vi "CSV_Setup_Data_Handler_2.0.vi"(0 "first iteration":bool, 1 "Timeout 1":bool, 7 "Sample Data":dbl[](array[numeric]), 9 "Sample Data 2":dbl[](array[numeric]), 11 "Data":T1={"Camera 1"={"Camera1"="", "Cam 1"=FALSE, "CAM1 Model"=enum."a2A5328-15ucBAS", "Cam1 ID"=0}, "Camera 2"={"Camera2"="", "Cam 2"=FALSE, "CAM2 Model"=enum."a2A5328-15ucBAS", "Cam2 ID"=0}, "Image"={"Camera1_Img"=refnum, "Camera2_Img"=refnum, "Img1_Orig_Disp"=refnum, "Img2_Orig_Disp"=refnum, "Img1_Orig_RGB"=refnum, "Img2_Orig_RGB"=refnum, "Blue_Plane_Extract"=refnum, "Subtracted_Plane"=refnum, "Img1_Binary"=refnum, "Img2_Binary"=refnum, "Crop_Mask"=refnum, "Img1_Save"=refnum, "Img2_Save"=refnum, "Img1_Cali_Full"=refnum, "Img2_Cali_Full"=refnum, "Img1_Cali_Detect"=refnum, "Img2_Cali_Detect"=refnum}, "Ques"={"Cam 1 queue"=refnum, "Cam 2 queue"=refnum, "Cam 1 - save queue"=refnum, "Cam 2 - save queue"=refnum, "Image Process Queue Size"=500, "Image Save Queue Size"=500, "Overload threshold"=500, "Max large object threshold"=0}, "Arduino SRS"={"Pinch-valve"="", "Actuator"=FALSE, "Arduino Uno"="", "Valve state"=enum."Open"}, "Pump"={"Port"="", "Connection"=FALSE, "Flush Size"=0, "Command"="", "Pump Size"=enum."Large", "Pump"="", "Ready"=FALSE}, "Camera settings"={"Detection settings"={"Sample size threshold"=500, "Detection Region %"=30.0, "Timeout Sample"=200}, "Lens/camera settings"={"Aperture"=enum."Item 0", "Legacy Cam Attributes"=FALSE, "Max Framerate"=100, "Exposure Time"=1000.0, "Framerate"=15}, "Crop settings"={"Cam1"={"Rectangle 1"={"Left"=0, "Top"=0, "Right"=0, "Bottom"=0, "Rotation"=0.0}, "Camera Orientation 1"="", "Pixel to mm 1"=0.0}, "Cam2"={"Rectangle 2"={"Left"=0, "Top"=0, "Right"=0, "Bottom"=0, "Rotation"=0.0}, "Camera Orientation 2"="", "Pixel to mm 2"=0.0}}}, "Arduino ISS"={"Mega F3"="", "Phase3"=FALSE, "Barcode"="", "Sorting sys."=FALSE, "Initial size"=0.0, "Size Interval"=0.0, "Mun. of containers"=0.0, "Container nr."=0.0, "Arduino Mega"="", "Attempts"=0.0}, "Img_Capt"=FALSE, "Empty_Refill"=FALSE, "I don't think is in use"={"Light intensity"=100}, "Extended setup"={"Location"="Station", "Latitude"="Station", "Longitude"="Station", "Determiner"="Station", "Sex"="Station", "Station"="", "Collection date"=""}, "Main interface"={"Sample Name"="Test Sample", "Operator"="JFR", "Species Name"="", "Other Notes"=""}, "Tap1"=0, "SystemVersion"=0, "System Serial"="", "Exit"=FALSE, "Kuvette Full"=FALSE, "Core JKI"={"Current VI Reference"=refnum, "Close Panel on Exit?"=FALSE}, "Calibration"={"Calibration 1"=path "C:/Users/au540322/Desktop/IHS_Project/images/Debris/Debris_0/Debris_0_2019_06_01-23-32-49-686.PNG", "Calibration 2"=path "C:/Users/au540322/Desktop/IHS_Project/images/Debris/Debris_0/Debris_0_2019_06_01-23-32-49-686.PNG", "Detect 1"=path "C:/Users/au540322/Desktop/IHS_Project/images/Debris/Debris_0/Debris_0_2019_06_01-23-32-49-686.PNG", "Detect 2"=path "C:/Users/au540322/Desktop/IHS_Project/images/Debris/Debris_0/Debris_0_2019_06_01-23-32-49-686.PNG"}, "Auto Flush"=FALSE, "Status History"="", "Timestamp Start"=""} {"SystemVersion" items=["Standard", "XL"]; "Tap1" items=["Session Data", "Extended Setup", "Buffer", "Camera", "Dispenser", "Stats", "Connections"]; "I don't think is in use"."Light intensity" scale=0.0..100.0; "Camera settings"."Crop settings"."Cam2"."Rectangle 2"."Rotation" format="%.2f"; "Camera settings"."Crop settings"."Cam2"."Rectangle 2"."Left" scale=0.0..1024.0; "Camera settings"."Crop settings"."Cam2"."Rectangle 2"."Right" scale=0.0..1024.0; "Camera settings"."Crop settings"."Cam1"."Rectangle 1"."Rotation" format="%.2f"; "Camera settings"."Crop settings"."Cam1"."Rectangle 1"."Left" scale=0.0..1024.0; "Camera settings"."Crop settings"."Cam1"."Rectangle 1"."Right" scale=0.0..1024.0; "Camera settings"."Lens/camera settings"."Framerate" min=1; "Camera settings"."Lens/camera settings"."Max Framerate" min=1; "Camera settings"."Detection settings"."Sample size threshold" min=1; "Pump"."Flush Size" min=0 max=6000 step=100; "Ques"."Overload threshold" min=1; "Ques"."Image Save Queue Size" min=1; "Ques"."Image Process Queue Size" min=1}, 12 "Timeout 2":bool) -> (4 "Sample Name":string, 6 "Ready file created":bool, 8 "Container num. Out":i32=2, 10 "Cam1_Stats":cluster{"Mean_Area":i32, "Img_Count":u32} caption="Camera 1", 14 "Container barcode":string, 15 "Cam2_Stats":cluster{"Mean_Area":i32, "Img_Count":u32} caption="Camera 2")   [LabVIEW 2024]
uses:
  controls/Data_JKI.ctl
  <vilib>/userDefined/High Color/IMAQdx.ctl
  <vilib>/vision/Image Controls.llb/IMAQ Image.ctl
panel:
  in  "Stop":bool
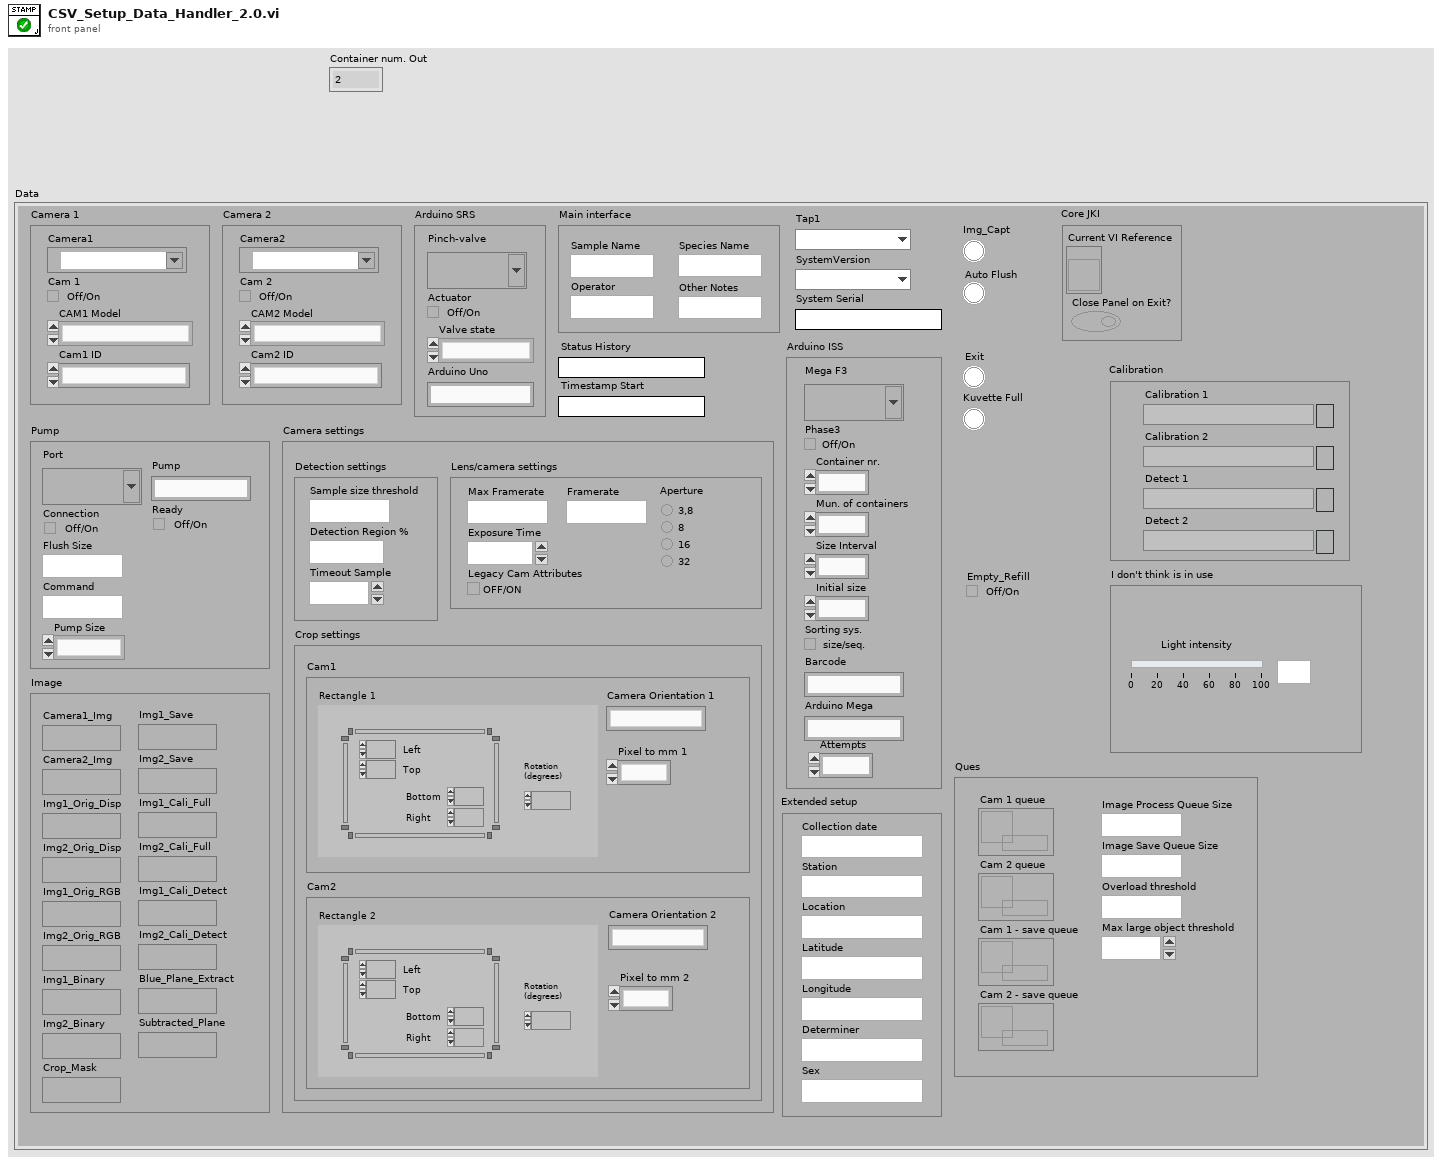
[diagram p1: front panel]
types:
  T1 = typedef "Data_JKI.ctl" = cluster{"Camera 1":cluster{"Camera1":T2, "Cam 1":bool, "CAM1 Model":enum16{"a2A5328-15ucBAS", "acA1920-155uc"}, "Cam1 ID":i32}, "Camera 2":cluster{"Camera2":T2, "Cam 2":bool, "CAM2 Model":enum16{"a2A5328-15ucBAS", "acA1920-155uc"}, "Cam2 ID":i32}, "Image":cluster{"Camera1_Img":T3, "Camera2_Img":T3, "Img1_Orig_Disp":T3, "Img2_Orig_Disp":T3, "Img1_Orig_RGB":T3, "Img2_Orig_RGB":T3, "Blue_Plane_Extract":T3, "Subtracted_Plane":T3, "Img1_Binary":T3, "Img2_Binary":T3, "Crop_Mask":T3, "Img1_Save":T3, "Img2_Save":T3, "Img1_Cali_Full":T3, "Img2_Cali_Full":T3, "Img1_Cali_Detect":T3, "Img2_Cali_Detect":T3}, "Ques":cluster{"Cam 1 queue":refnum<queue>, "Cam 2 queue":refnum<queue>, "Cam 1 - save queue":refnum<queue>, "Cam 2 - save queue":refnum<queue>, "Image Process Queue Size":i32, "Image Save Queue Size":i32, "Overload threshold":i32, "Max large object threshold":i32}, "Arduino SRS":cluster{"Pinch-valve":refnum<visa-resource-name>, "Actuator":bool, "Arduino Uno":string, "Valve state":enum16{"Standby", "Close", "Open"}}, "Pump":cluster{"Port":refnum<visa-resource-name>, "Connection":bool, "Flush Size":i32, "Command":string, "Pump Size":enum16{"None", "Small", "Large"}, "Pump":string, "Ready":bool}, "Camera settings":cluster{"Detection settings":cluster{"Sample size threshold":i32, "Detection Region %":dbl, "Timeout Sample":i32}, "Lens/camera settings":cluster{"Aperture":enum32{"Item 0", "Item 1", "Item 2", "Item 3"}, "Legacy Cam Attributes":bool, "Max Framerate":i32, "Exposure Time":dbl, "Framerate":i32}, "Crop settings":cluster{"Cam1":cluster{"Rectangle 1":T4, "Camera Orientation 1":string, "Pixel to mm 1":dbl}, "Cam2":cluster{"Rectangle 2":T4, "Camera Orientation 2":string, "Pixel to mm 2":dbl}}}, "Arduino ISS":cluster{"Mega F3":refnum<visa-resource-name>, "Phase3":bool, "Barcode":string, "Sorting sys.":bool, "Initial size":dbl, "Size Interval":dbl, "Mun. of containers":dbl, "Container nr.":dbl, "Arduino Mega":string, "Attempts":dbl}, "Img_Capt":bool, "Empty_Refill":bool, "I don't think is in use":cluster{"Light intensity":i32}, "Extended setup":cluster{"Location":string, "Latitude":string, "Longitude":string, "Determiner":string, "Sex":string, "Station":string, "Collection date":string}, "Main interface":cluster{"Sample Name":string, "Operator":string, "Species Name":string, "Other Notes":string}, "Tap1":u16, "SystemVersion":u16, "System Serial":string, "Exit":bool, "Kuvette Full":bool, "Core JKI":cluster{"Current VI Reference":refnum<vi>, "Close Panel on Exit?":bool}, "Calibration":cluster{"Calibration 1":path, "Calibration 2":path, "Detect 1":path, "Detect 2":path}, "Auto Flush":bool, "Status History":string, "Timestamp Start":string}
  T2 = typedef "IMAQdx.ctl" = refnum<k21>
  T3 = typedef "IMAQ Image.ctl" = refnum<image>
  T4 = typedef "IMAQ Rectangle" = cluster{"Left":i32, "Top":i32, "Right":i32, "Bottom":i32, "Rotation":dbl}
  T5 = cluster{"MFD max":string, "MFD mean":string, "MFD std. dev.":string, "Perim. mean":string, "Perim. std. dev":string, "Area mean":string, "Area std. dev.":string, "Holes mean":string, "Holes std. dev.":string, "Area+Holes mean":string, "Area+Holes std. dev.":string}
  T6 = cluster{"MFD max":string, "MFD mean":string, "MFD std. dev.":string, "Perim. mean":string, "Perim. std. dev":string, "Area mean":string, "Area std. dev.":string, "Holes mean":string, "Holes std. dev.":string, "Area+Holes mean":string, "Area+Holes std. dev.":string, "Barcode":string}
  T7 = cluster{"MFD max":string, "MFD mean":string, "MFD std. dev.":string, "Perim. mean":string, "Perim. std. dev":string, "Area mean":string, "Area std. dev.":string, "Holes mean":string, "Holes std. dev.":string, "Area+Holes mean":string, "Area+Holes std. dev.":string, "Container barcode":string}
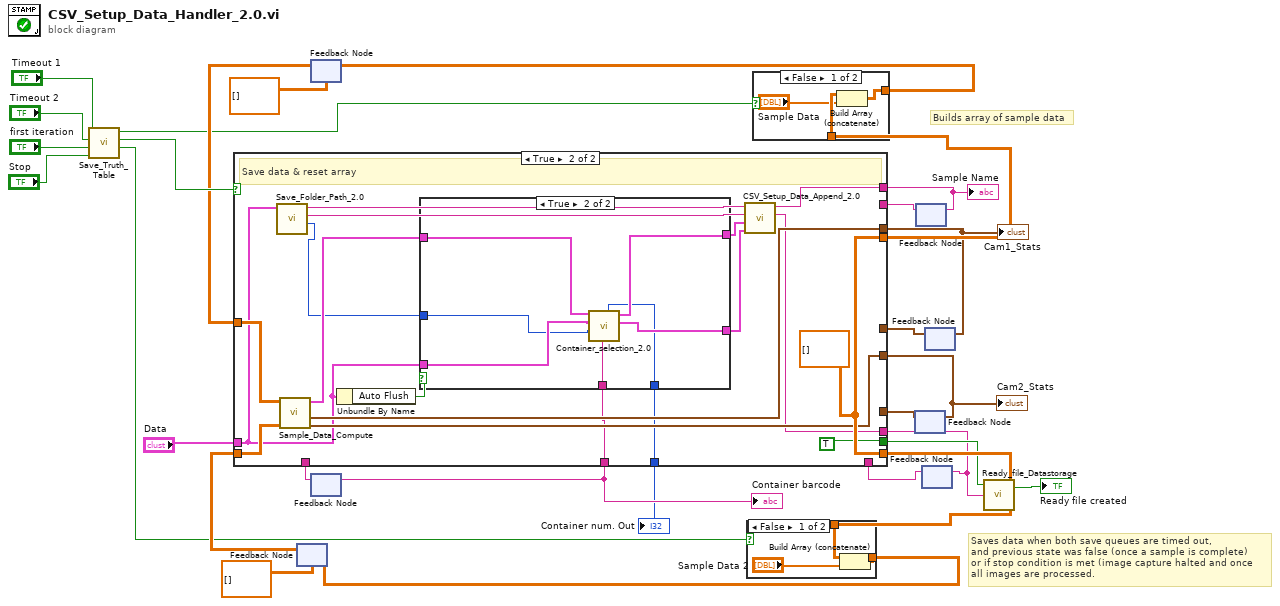
[diagram p0: block diagram]
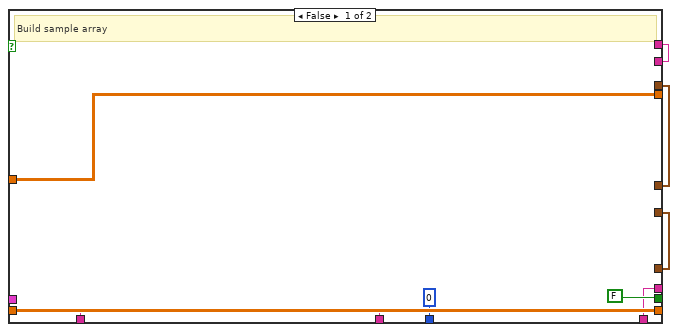
[diagram p4: hidden frame]
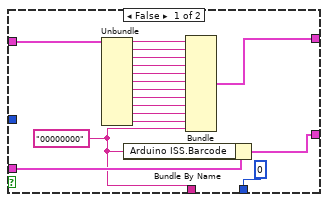
[diagram p5: hidden frame]
diagram:
  # "Builds array of sample data"
  # "Saves data when both save queues are timed out, \nand previous state was false (once a sample is complete)\nor if stop condition is met (image capture halted and once\nall images are processed."
  n1 = call "Save_Truth_Table.vi"("Stop"="Stop", "first iteration"="first iteration", "Timeout 2"="Timeout 2", "Timeout 1"="Timeout 1") -> ("Append Sample Data 2"=w19:bool, "Save_Data"=w22:bool, "Append Sample Data 1"=w20:bool)  [unwired: 5 in]
  n2 = feedback #1(dbl[][] []) -> (w25:dbl[][])
  n3 = feedback #2(dbl[][] []) -> (w21:dbl[][])
  n4 = feedback #3() -> (w3:string)  [unwired: 1 in]
  n5 = feedback #4() -> (w11:cluster{"Mean_Area":i32, "Img_Count":u32})  [unwired: 1 in]
  n6 = feedback #5() -> (w13:string)  [unwired: 1 in]
  n7 = feedback #6() -> (w6:string)  [unwired: 1 in]
  n8 = feedback #7() -> (w12:cluster{"Mean_Area":i32, "Img_Count":u32})  [unwired: 1 in]
  n9 = case shown="True" w22 {
    tunnel: "Data" -> [_ w47]
    tunnel: w25 -> [w38 w55]
    tunnel: [w38 w56] -> w23
    tunnel: w21 -> [w37 w54]
    tunnel: [w37 w56] -> w29
    tunnel: [w36 w40] -> w14
    tunnel: [w34 w53] -> w10
    tunnel: [w35 w52] -> w9
    tunnel: w13 -> [w36 _]
    tunnel: w12 -> [w35 _]
    tunnel: w11 -> [w34 _]
    tunnel: [FALSE TRUE] -> w8
    tunnel: [w32 w41] -> w7
    tunnel: w6 -> [w32 _]
    tunnel: [w31 w49] -> w4
    tunnel: w3 -> [w31 _]
    tunnel: [0 ("Container num. Out") w39] -> w1
    frame False {
      # "Build sample array"
    }
    frame True {
      w56 = dbl[][] []
      # "Save data & reset array"
      n10 = call "Save_Folder_Path_2.0.vi"("Data"=w47) -> ("Sample cnt."=w46:i32, "Subfolder Name"=w44:string, "Subfolder Path"=w45:string)  [unwired: 8 in]
      n11 = call "Sample_Data_Compute.vi"("Data Array 2"=w55, "Data Array 1"=w54) -> ("Cam2_Stats"=w53:cluster{"Mean_Area":i32, "Img_Count":u32}, "Cam1_Stats"=w52:cluster{"Mean_Area":i32, "Img_Count":u32}, "output cluster"=w50:T5)  [unwired: 6 in, 1 out]
      n12 = Unbundle By Name(w47) -> ("Auto Flush"=w48:bool)
      n13 = case shown="True" w48 {
        tunnel: [w72 w76] -> w42
        tunnel: w50 -> [w71 w80]
        tunnel: [w58 w75] -> w43
        tunnel: [w59 w77] -> w49
        tunnel: w46 -> [_ w78]
        tunnel: w47 -> [w73 w79]
        tunnel: [0 ("Container num. Out") w74] -> w39
        frame False {
          w59 = "00000000" ("Barcode")
          n14 = Unbundle(w71) -> ("MFD max"=w70:string, "MFD mean"=w69:string, "MFD std. dev."=w68:string, "Perim. mean"=w67:string, "Perim. std. dev"=w66:string, "Area mean"=w65:string, "Area std. dev."=w64:string, "Holes mean"=w63:string, "Holes std. dev."=w62:string, "Area+Holes mean"=w61:string, "Area+Holes std. dev."=w60:string)
          n15 = Bundle By Name(cluster=w73, "Arduino ISS.Barcode"=w59) -> (w72:T1)
          n16 = Bundle("MFD max"=w70, "MFD mean"=w69, "MFD std. dev."=w68, "Perim. mean"=w67, "Perim. std. dev"=w66, "Area mean"=w65, "Area std. dev."=w64, "Holes mean"=w63, "Holes std. dev."=w62, "Area+Holes mean"=w61, "Area+Holes std. dev."=w60, "Barcode"=w59) -> (w58:T6)  [unwired: 1 in]
        }
        frame True {
          n17 = call "Container_selection_2.0.vi"("Insect number"=w78, "Data"=w79, "Input cluster"=w80) -> ("output cluster 2"=w76:T1, "output cluster"=w75:T7, "Container num. Out"=w74:i32, "Container barcode"=w77:string)  [unwired: 2 in, 3 out]
        }
      }
      n18 = call "CSV_Setup_Data_Append_2.0.vi"("Data"=w42, "Sample cluster"=w43, "Sample Name"=w44, "Image path"=w45) -> ("File Path"=w41:string, "Sample Name dup"=w40:string)  [unwired: 6 in]
    }
  }
  "Sample Name" <- w14
  "Cam1_Stats" <- w9
  "Cam2_Stats" <- w10
  "Container barcode" <- w4
  "Container num. Out" <- w1
  n19 = feedback-in #3(w4) -> ()
  n20 = case shown="False" w19 {
    tunnel: [w83 w84] -> w24
    tunnel: w23 -> [w82 w84]
    frame False {
      n21 = Build Array (concatenate)(w82, "Sample Data 2") -> (w83:dbl[][])
    }
    frame True {
    }
  }
  n22 = feedback-in #1(w24) -> ()
  n23 = case shown="False" w20 {
    tunnel: w29 -> [w87 w88]
    tunnel: [w86 w88] -> w26
    frame False {
      n24 = Build Array (concatenate)(w87, "Sample Data") -> (w86:dbl[][])
    }
    frame True {
    }
  }
  n25 = feedback-in #2(w26) -> ()
  n26 = feedback-in #4(w10) -> ()
  n27 = feedback-in #5(w14) -> ()
  n28 = feedback-in #6(w7) -> ()
  n29 = feedback-in #7(w9) -> ()
  n30 = call "Ready_file_Datastorage.vi"("File Path"=w7, "File save"=w8) -> ("Ready file created"=→"Ready file created":bool)  [unwired: 2 in]
